vi "Main.vi"() -> ()   [LabVIEW 2020]
doc: "Elevator CLA examen is base on QMH and event for communication \nXML for database"
uses:
  controls/FGV_To_Do.ctl
panel:
  in  "error in (no error)":errorcluster
types:
  T1 = typedef "FGV_To_Do.ctl" = enum16{"1 - Initialize_Events", "2 - Read_Database", "3 - Initialize QMH", "Save_Database", "Read", "4 - Close_Events", "5 - Close_QMH"}
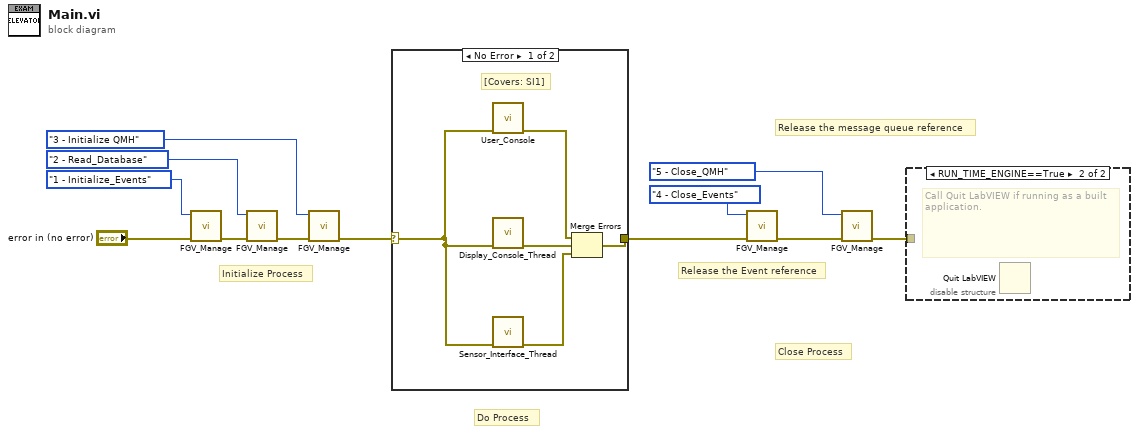
[diagram p0: block diagram]
diagram:
  # "Do Process"
  # "Close Process"
  # "Initialize Process"
  # "Release the Event reference"
  # "Release the message queue reference"
  n1 = call "FGV_Manage.vi"("error in (no error)"="error in (no error)", "To do"=FGV_To_Do."1 - Initialize_Events") -> ("error out"=w4:errorcluster)  [unwired: 8 in, 1 out]
  n2 = call "FGV_Manage.vi"("error in (no error)"=w4, "To do"=FGV_To_Do."2 - Read_Database") -> ("error out"=w3:errorcluster)  [unwired: 8 in, 1 out]
  n3 = call "FGV_Manage.vi"("error in (no error)"=w3, "To do"=FGV_To_Do."3 - Initialize QMH") -> ("error out"=w2:errorcluster)  [unwired: 8 in, 1 out]
  n4 = case shown="No Error" w2 {
    selector: w2 -> [w14 w18]
    tunnel: [w16 w18] -> w9
    frame No Error {
      # "[Covers: SI1]"
      n5 = call "User_Console.vi"("error in (no error)"=w14) -> ("error out"=w17:errorcluster)  [unwired: 10 in]
      n6 = call "Display_Console_Thread.vi"("error in (no error)"=w14) -> ("error out"=w15:errorcluster)  [unwired: 10 in]
      n7 = call "Sensor_Interface_Thread.vi"("error in (no error)"=w14) -> ("error out"=w13:errorcluster)  [unwired: 10 in]
      n8 = Merge Errors(w17, w15, w13) -> (w16:errorcluster)
    }
    frame Error {
    }
  }
  n9 = call "FGV_Manage.vi"("error in (no error)"=w9, "To do"=FGV_To_Do."4 - Close_Events") -> ("error out"=w7:errorcluster)  [unwired: 8 in, 1 out]
  n10 = call "FGV_Manage.vi"("error in (no error)"=w7, "To do"=FGV_To_Do."5 - Close_QMH") -> ("error out"=w6:errorcluster)  [unwired: 8 in, 1 out]
  n11 = disable-structure shown="RUN_TIME_ENGINE==True" {
    disable-tunnel: w6 -> [_ _]
    frame condition #0 (active) {
    }
    frame condition #1 {
      # "Call Quit LabVIEW if running as a built application."
      n12 = Quit LabVIEW() -> ()  [unwired: 1 in]
    }
  }
